vi "UI.vi"(8 "error in (no error)":errorcluster, 9 "timeout":bool, 10 "_data.lvlib:_data.lvclass":refnum<class "_data.lvclass">, 11 "dataTA in":refnum<class "dataTA.lvclass">) -> (0 "error out":errorcluster, 3 "dataTA out":refnum<class "dataTA.lvclass">)   [LabVIEW 2019, in "dataTA.lvlib" / "dataTA.lvclass"]
uses:
  dataTA.lvclass
  _data/_data.lvlibp/_dataClass/_data.lvclass
panel:
  in  "Tab Control":enum32{"Page 1", "Page 2"}(tab)
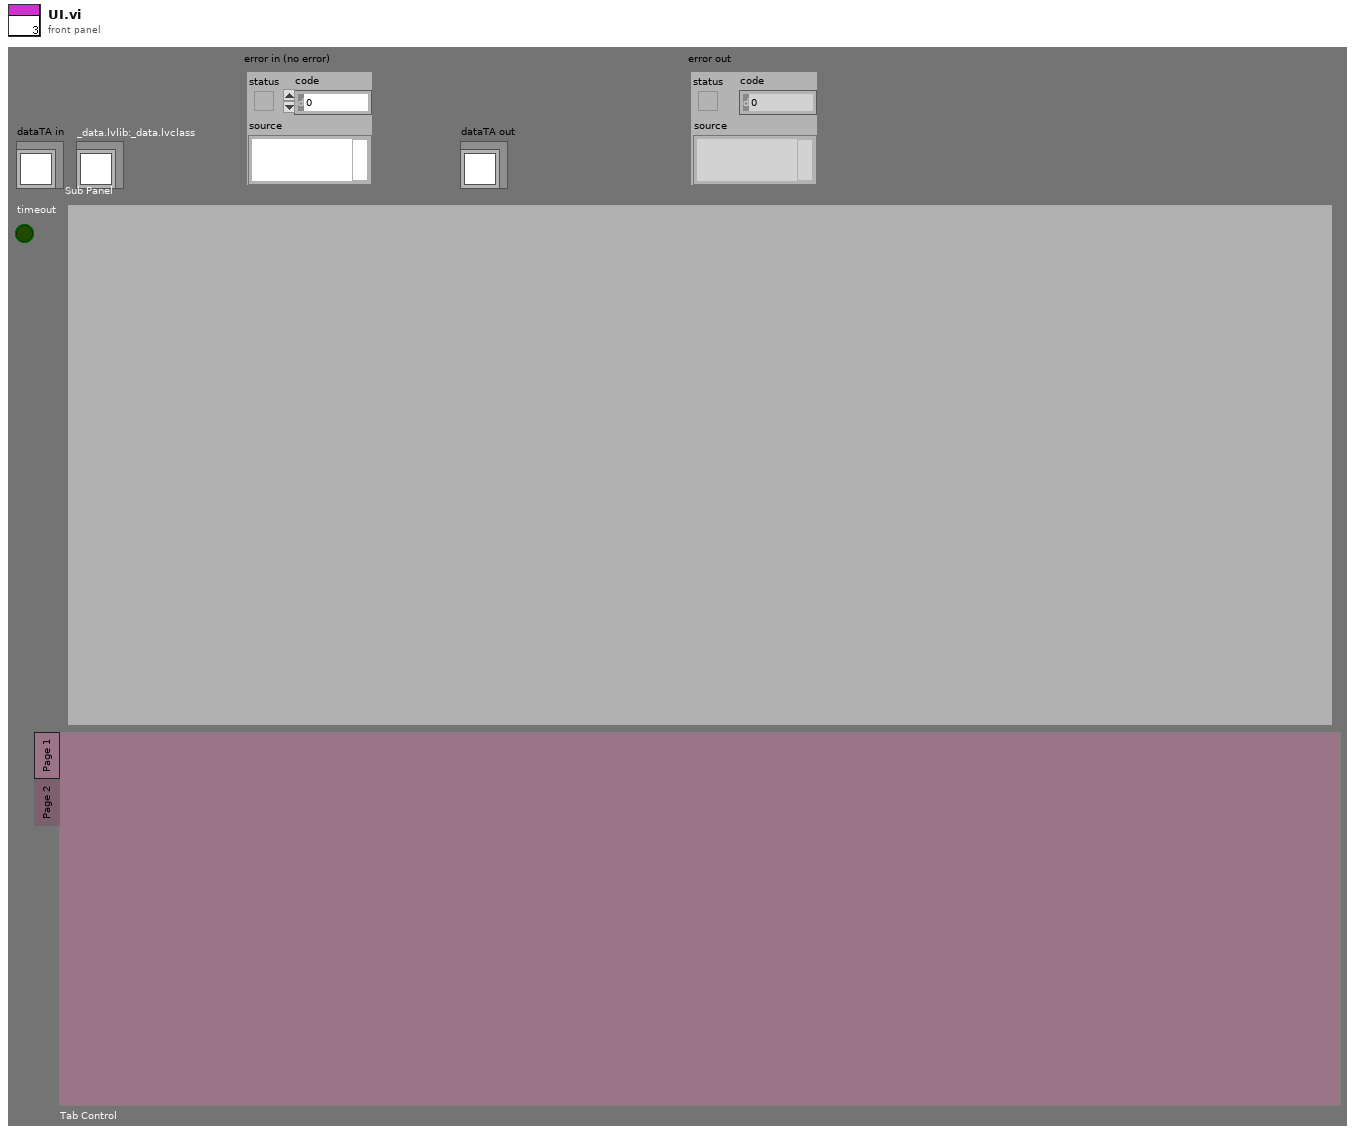
[diagram p1: front panel]
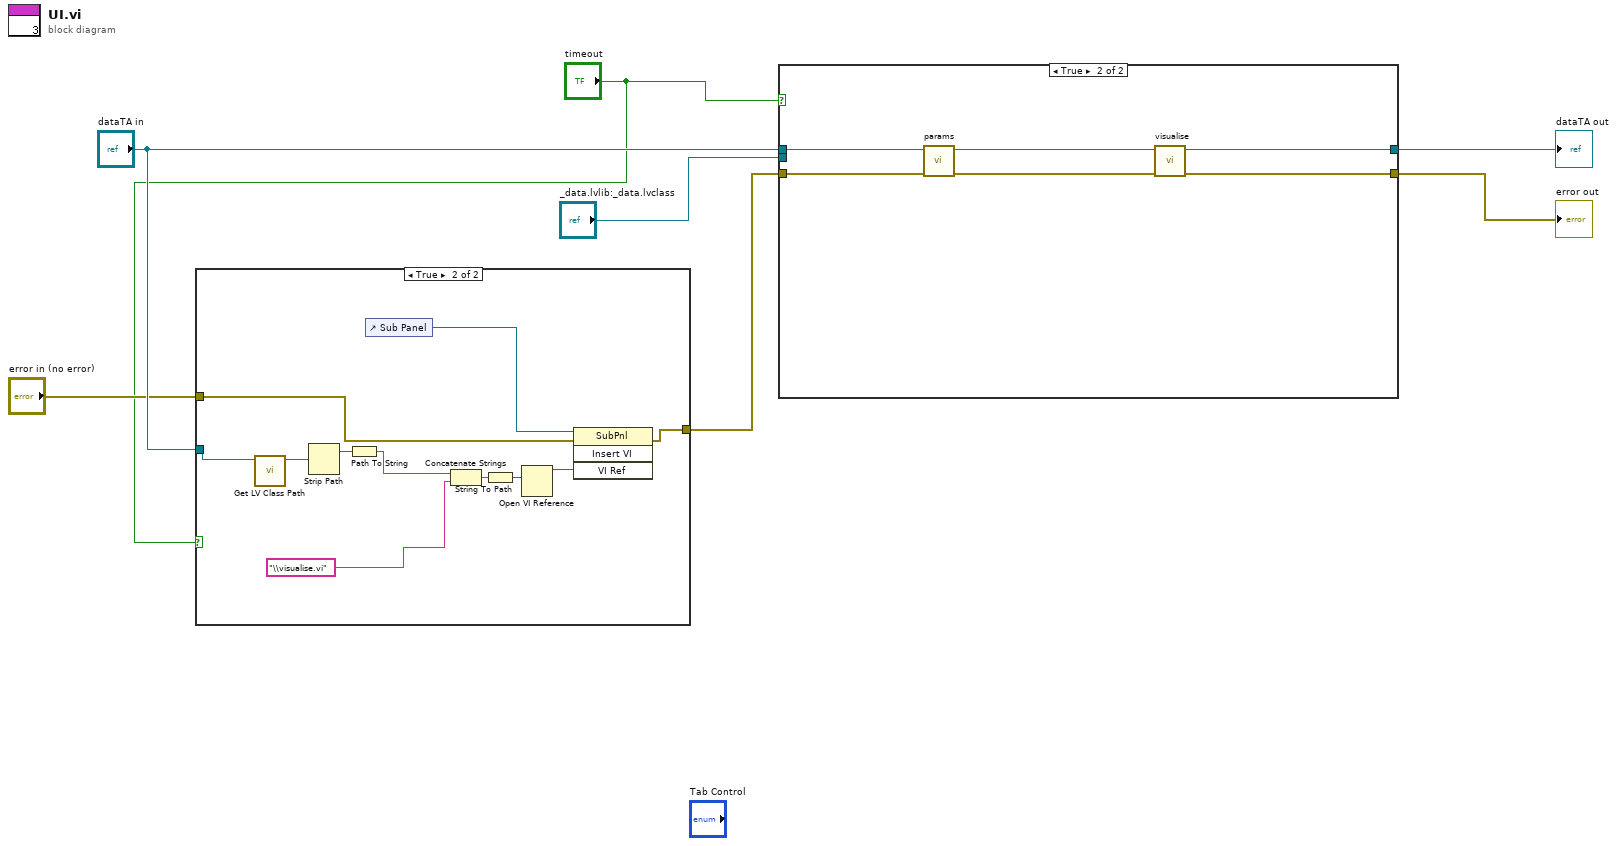
[diagram p0: block diagram]
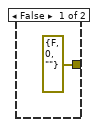
[diagram p2: hidden frame]
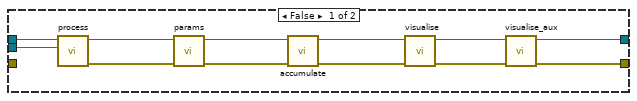
[diagram p3: hidden frame]
diagram:
  n1 = case shown="True" "timeout" {
    tunnel: [errorcluster {"status"=FALSE, "code"=0, "source"=""} ("error out") w19] -> w4
    tunnel: "dataTA in" -> [_ w18]
    tunnel: "error in (no error)" -> [_ w9]
    frame False {
    }
    frame True {
      n2 = call <vilib>:"Get LV Class Path.vi"("object"=w18) -> ("class path"=w13:path)  [unwired: 9 in, 1 out]
      n3 = Strip Path(path=w13) -> (stripped path=w12:path)  [unwired: 1 out]
      n4 = Path To String(path=w12) -> (string=w11:string)
      n5 = control-ref of="Sub Panel"() -> (w17:refnum<vi>)
      n6 = Concatenate Strings(w11, "\\visualise.vi" ("string")) -> (w14:string)
      n7 = String To Path(string=w14) -> (path=w15:path)
      n8 = Open VI Reference(vi path=w15) -> (vi reference=w10:refnum<vi>)  [unwired: 5 in, 1 out]
      n9 = invoke class="SubPnl" method="Insert VI"(reference=w17, error in=w9, "VI Ref"=w10) -> (error out=w19:errorcluster)  [unwired: 1 in, 3 out]
    }
  }
  n10 = case shown="True" "timeout" {
    tunnel: "dataTA in" -> [w31 w37]
    tunnel: [w26 w33] -> w7
    tunnel: "_data.lvlib:_data.lvclass" -> [w25 _]
    tunnel: [w20 w34] -> w5
    tunnel: w4 -> [_ w32]
    frame False {
      n11 = call-dynamic "process.vi"("_data.lvlibp:_data.lvclass"=w25, "dataTA in"=w31) -> ("error out"=w24:errorcluster, "dataTA out"=w30:refnum<class "dataTA.lvclass">)  [unwired: 8 in]
      n12 = call-dynamic "params.vi"("error in (no error)"=w24, "dataTA in"=w30) -> ("error out"=w23:errorcluster, "dataTA out"=w29:refnum<class "dataTA.lvclass">)  [unwired: 8 in]
      n13 = call-dynamic "accumulate.vi"("error in (no error)"=w23, "dataTA in"=w29) -> ("error out"=w22:errorcluster, "dataTA out"=w28:refnum<class "dataTA.lvclass">)  [unwired: 8 in]
      n14 = call-dynamic "visualise.vi"("error in (no error)"=w22, "dataTA in"=w28) -> ("error out"=w21:errorcluster, "dataTA out"=w27:refnum<class "dataTA.lvclass">)  [unwired: 8 in]
      n15 = call-dynamic "visualise_aux.vi"("error in (no error)"=w21, "dataTA in"=w27) -> ("error out"=w20:errorcluster, "dataTA out"=w26:refnum<class "dataTA.lvclass">)  [unwired: 8 in]
    }
    frame True {
      n16 = call-dynamic "params.vi"("error in (no error)"=w32, "dataTA in"=w37) -> ("error out"=w36:errorcluster, "dataTA out"=w35:refnum<class "dataTA.lvclass">)  [unwired: 8 in]
      n17 = call-dynamic "visualise.vi"("error in (no error)"=w36, "dataTA in"=w35) -> ("error out"=w34:errorcluster, "dataTA out"=w33:refnum<class "dataTA.lvclass">)  [unwired: 8 in]
    }
  }
  "error out" <- w5
  "dataTA out" <- w7
